vi "Test Properties Report (Events).vi"() -> ()   [LabVIEW 2013]
uses:
  classes/Test Suite/Test Suite.lvclass
  classes/Test Report.Event/Test Report.Event.lvclass
panel:
  out "individual assertion events":string
  out "final report":string
  in  "error in (no error)":errorcluster
  out "error out":errorcluster
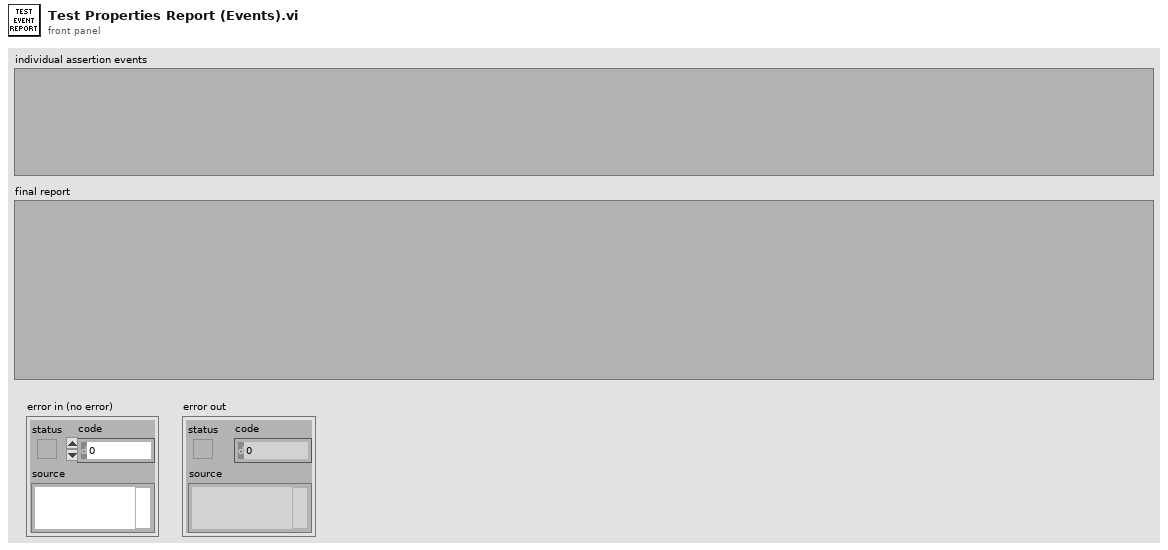
[diagram p1: front panel]
types:
  T1 = typedef "Caraya.lvlib/Test Suite.lvclass/Suite PublicEvents -- cluster.ctl" = cluster{"Test Suite Result Event":refnum<user-event>, "suite destroyed":refnum<user-event>, "Test Registration Event":refnum<user-event>, "Assertion Event":refnum<user-event>, "Assertion Update Event":refnum<user-event>}
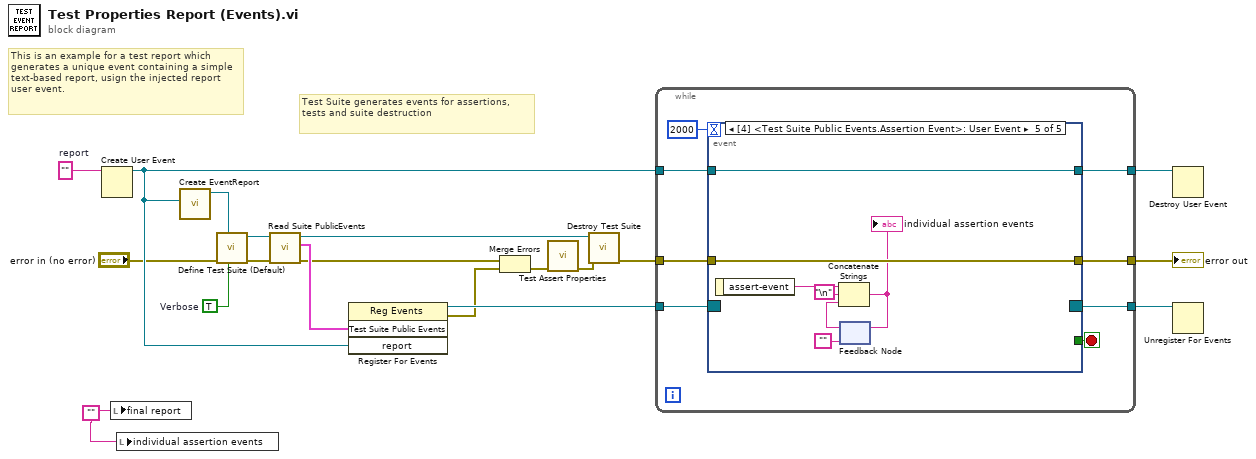
[diagram p0: block diagram]
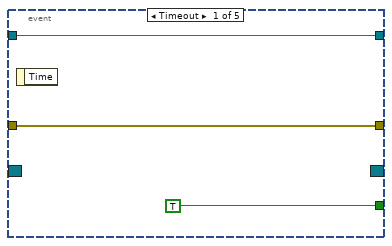
[diagram p2: hidden frame]
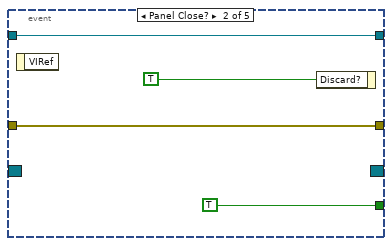
[diagram p3: hidden frame]
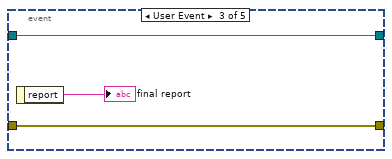
[diagram p4: hidden frame]
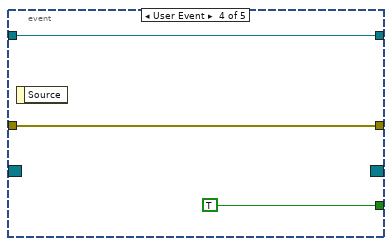
[diagram p5: hidden frame]
diagram:
  w1 = ""
  w16 = ""  # report
  w17 = TRUE  # Verbose
  # "Test Suite generates events for assertions, tests and suite destruction"
  # "This is an example for a test report which generates a unique event containing a simple text-based report, usign the injected report user event."
  n1 = Create User Event(user event datatype=w16) -> (user event=w8:refnum<user-event>)  [unwired: 1 in, 1 out]
  n2 = local write "final report"(w1) -> ()
  n3 = local write "individual assertion events"(w1) -> ()
  n4 = call "Create EventReport.vi"("Report Event"=w8) -> ("Test Report.Event out"=w18:refnum<class "Test Report.Event.lvclass">)  [unwired: 9 in, 1 out]
  n5 = call "Define Test Suite (Default).vi"("Verbose (F)"=w17, "Test Report (optional)"=w18, "error in (no error)"="error in (no error)") -> ("error out"=w9:errorcluster, "Test Suite"=w11:refnum<class "Test Suite.lvclass">)  [unwired: 6 in, 1 out]
  n6 = call "Read Suite PublicEvents.vi"("error in (no error)"=w9, "Test Suite in"=w11) -> ("error out"=w4:errorcluster, "Test Suite Public Events"=w5:T1, "Test Suite out"=w10:refnum<class "Test Suite.lvclass">)  [unwired: 7 in]
  n7 = register-events(w5, w8) -> (reference out=w7:refnum<event-registration>, error out=w3:errorcluster)  [unwired: 2 in]
  n8 = Merge Errors(w4, w3) -> (w2:errorcluster)
  n9 = call "Test Assert Properties.vi"("error in (no error)"=w2) -> ("error out"=w19:errorcluster)  [unwired: 10 in]
  n10 = call-dynamic "Destroy Test Suite.vi"("error in (no error)"=w19, "Test Suite in"=w10) -> ("error out"=w13:errorcluster)  [unwired: 8 in, 1 out]
  n11 = while {
    tunnel: [w27] -> w15
    tunnel: [w26] -> w14
    tunnel: w13 -> [w24]
    tunnel: [w23] -> w12
    tunnel: w8 -> [w22]
    tunnel: w7 -> [w21]
    stop <- w20 stop-if-true
    n12 = event shown="[4] <Test Suite Public Events.Assertion Event>: User Event" {
      selector: w21 -> [_ _ _ _ _]
      dyn-events: [_ _ _ _ _] -> w27
      timeout: 2000 -> [_ _ _ _ _]
      tunnel: [w30 w34 w37 w38 w47] -> w26
      tunnel: w22 -> [w30 w34 w37 w38 w47]
      tunnel: w24 -> [w29 w32 w36 w39 w46]
      tunnel: [w29 w32 w36 w39 w46] -> w23
      tunnel: [TRUE TRUE _ TRUE _] -> w20
      event Timeout {
        n13 = event-data() -> ()  [unwired: 1 in, 1 out]
      }
      event Panel Close? {
        n14 = event-data() -> ()  [unwired: 1 in, 1 out]
        n15 = event-data("Discard?"=TRUE) -> ()  [unwired: 1 in, 1 out]
      }
      event User Event {
        n16 = event-data() -> ("report"=→"final report":string)  [unwired: 1 in]
      }
      event User Event {
        n17 = event-data() -> ()  [unwired: 1 in, 1 out]
      }
      event User Event {
        n18 = event-data() -> ("assert-event"=w45:string)  [unwired: 1 in]
        n19 = feedback #1("") -> (w44:string)
        n20 = Concatenate Strings(w45, "\n", w44) -> (w41:string)
        "individual assertion events" <- w41
        n21 = feedback-in #1(w41) -> ()
      }
    }
  }
  "error out" <- w12
  n22 = Destroy User Event(user event=w14) -> ()  [unwired: 1 in, 1 out]
  n23 = Unregister For Events(event registration refnum=w15) -> ()  [unwired: 1 in, 1 out]
